vi "Spectral Save Queue.vi"(4 "timeout in ms (-1)":i32=10, 6 "max queue size (-1, unlimited)":i32, 7 "Action":T1=enum."Enqueue", 8 "error in (no error)":errorcluster, 11 "data in":u16[][](array[numeric])) -> (0 "error out":errorcluster, 1 "Empty?":bool, 2 "# elements in queue":i32, 3 "data out":u16[][](array[numeric]))   [LabVIEW 2018]
uses:
  Controls/Queue Manager Actions.ctl
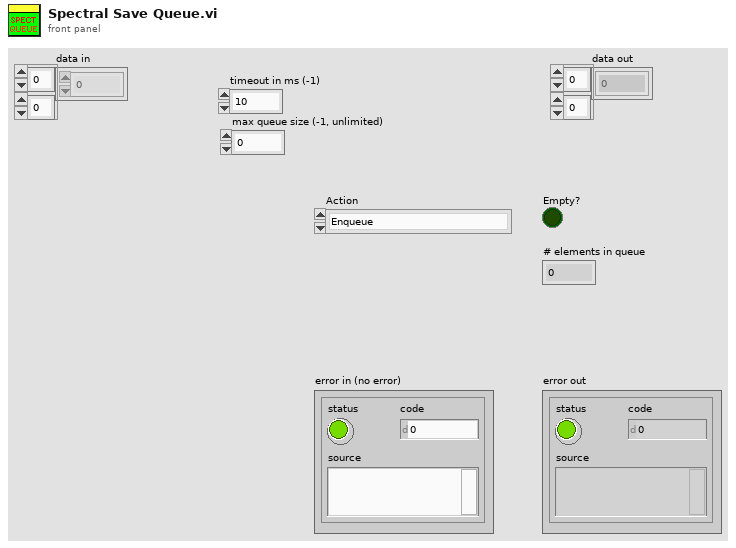
[diagram p1: front panel]
types:
  T1 = typedef "Queue Manager Actions.ctl" = enum16{"Init", "Enqueue", "Enqueue All", "Preview Queue", "Dequeue", "Get Status", "Flush Queue", "Flush All Queues", "Release All Queues", "Release Queue", "Enqueue at Opposite End"}
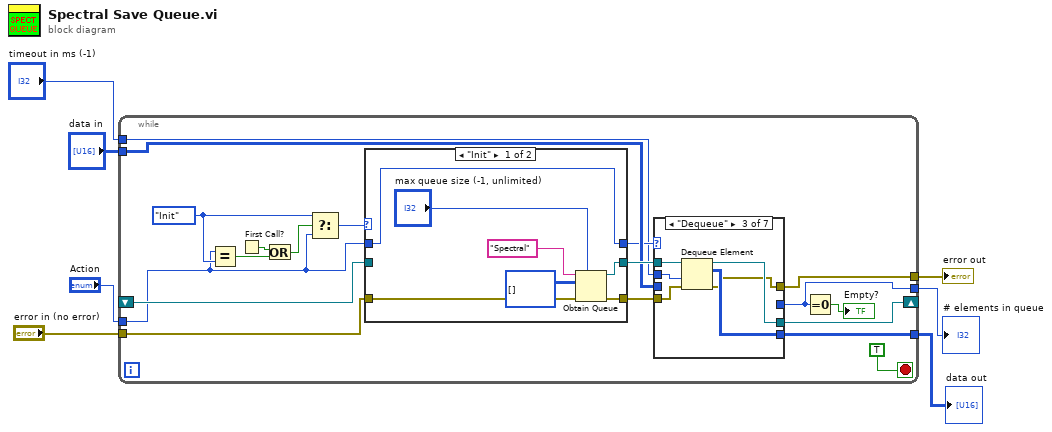
[diagram p0: block diagram]
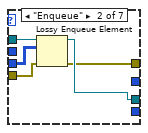
[diagram p3: hidden frame]
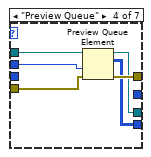
[diagram p4: hidden frame]
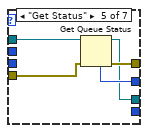
[diagram p5: hidden frame]
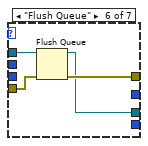
[diagram p6: hidden frame]
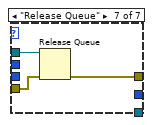
[diagram p7: hidden frame]
diagram:
  n1 = while {
    tunnel: "Action" -> [w9]
    tunnel: "error in (no error)" -> [w14]
    shift-right: [w16] -> _
    shift-left: _ -> [w15]
    tunnel: "data in" -> [w12]
    tunnel: "timeout in ms (-1)" -> [w8]
    tunnel: [w19] -> w3
    tunnel: [w18] -> w2
    tunnel: [w11] -> w1
    stop <- TRUE stop-if-true
    w21 = Queue_Manager_Actions."Init"
    n2 = Equal?(x=w9, y=w21) -> (x = y?=w23:bool)
    n3 = First Call?() -> (First Call?: T/F=w24:bool)
    n4 = Or(x=w24, y=w23) -> (x .or. y?=w22:bool)
    n5 = Select(t=w21, s=w22, f=w9) -> (s? t:f=w20:T1)
    n6 = case shown="\"Init\"" w20 {
      tunnel: [w64 w67] -> w17
      tunnel: [w63 w66] -> w13
      tunnel: w15 -> [_ w67]
      tunnel: w14 -> [w61 w66]
      tunnel: [w59 w65] -> w10
      tunnel: w9 -> [w59 w65]
      frame "Init" {
        n7 = Obtain Queue(max queue size (-1, unlimited)="max queue size (-1, unlimited)", name (unnamed)="Spectral", element data type=u16[][] [], error in (no error)=w61) -> (queue out=w64:refnum<queue>, error out=w63:errorcluster)  [unwired: 1 in, 1 out]
      }
      frame Default {
      }
    }
    n8 = case shown="\"Dequeue\"" w10 {
      tunnel: [w27 w29 w34 w45 w50 w54 w57] -> w19
      tunnel: [_ _ w39 w44 _ _ _] -> w18
      tunnel: [_ _ _ _ w49 _ _] -> w11
      tunnel: w17 -> [w28 w33 w38 w42 w48 w53 w56]
      tunnel: [w28 w30 w35 w41 w46 w51 _] -> w16
      tunnel: w13 -> [w27 w32 w37 w43 w47 w52 w55]
      tunnel: w12 -> [_ w31 _ _ _ _ _]
      tunnel: w8 -> [_ _ w36 w40 _ _ _]
      frame "Init", Default {
      }
      frame "Enqueue" {
        n9 = Lossy Enqueue Element(queue=w33, element=w31, error in (no error)=w32) -> (queue out=w30:refnum<queue>, error out=w29:errorcluster)  [unwired: 2 out]
      }
      frame "Dequeue" {
        n10 = Dequeue Element(queue=w38, timeout in ms (-1)=w36, error in (no error)=w37) -> (queue out=w35:refnum<queue>, element=w39:u16[][], error out=w34:errorcluster)  [unwired: 1 out]
      }
      frame "Preview Queue" {
        n11 = Preview Queue Element(queue=w42, timeout in ms (-1)=w40, error in (no error)=w43) -> (queue out=w41:refnum<queue>, element=w44:u16[][], error out=w45:errorcluster)  [unwired: 1 out]
      }
      frame "Get Status" {
        n12 = Get Queue Status(queue=w48, error in (no error)=w47) -> (queue out=w46:refnum<queue>, error out=w50:errorcluster, # elements in queue=w49:i32)  [unwired: 1 in, 5 out]
      }
      frame "Flush Queue" {
        n13 = Flush Queue(queue=w53, error in (no error)=w52) -> (queue out=w51:refnum<queue>, error out=w54:errorcluster)  [unwired: 1 out]
      }
      frame "Release Queue" {
        n14 = Release Queue(queue=w56, error in (no error)=w55) -> (error out=w57:errorcluster)  [unwired: 1 in, 2 out]
      }
    }
    n15 = Equal To 0?(x=w11) -> (x = 0?=→"Empty?":bool)
  }
  "error out" <- w3
  "# elements in queue" <- w1
  "data out" <- w2
